vi "Is Deserializer Resource.vi"(0 "serdes resource name":string) -> (4 "is deserializer resource":bool)   [LabVIEW 2023, in "GettingStarted_Common_148X_Host.lvlib"]
uses:
  GettingStarted_Common_148X_Host.lvlib
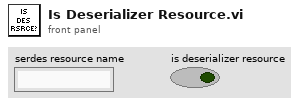
[diagram p1: front panel]
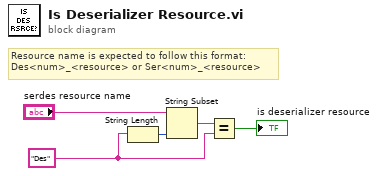
[diagram p0: block diagram]
diagram:
  w4 = "Des" ("y")
  # "Resource name is expected to follow this format: \nDes<num>_<resource> or Ser<num>_<resource>"
  n1 = String Length(string=w4) -> (length=w3:i32)
  n2 = String Subset(string="serdes resource name", length (rest)=w3) -> (substring=w2:string)  [unwired: 1 in]
  n3 = Equal?(x=w2, y=w4) -> (x = y?=→"is deserializer resource":bool)
